vi "EMG_Contraction_Detection.vi"(4 "Triceps EMG signal (V)":dbl[](array[numeric]), 6 "Biceps EMG signal (V)":dbl[](array[numeric]), 7 "Biceps contraction threshold (V)":dbl, 9 "Biceps harder contraction threshold  (V)":dbl, 10 "Triceps harderd contraction threshold  (V)":dbl, 11 "Triceps contraction threshold  (V)":dbl) -> (0 "Triceps mean amplitude during contraction  (V)":dbl, 1 "Triceps hardly contracted?":bool, 2 "Triceps contracted?":bool, 3 "Biceps contracted?":bool, 5 "Biceps hardly contracted?":bool, 8 "Biceps mean amplitude during contraction  (V)":dbl)   [LabVIEW 2015]
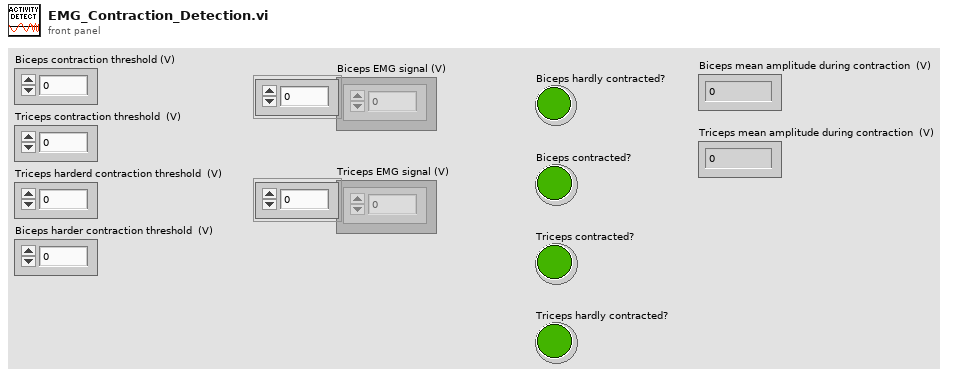
[diagram p1: front panel]
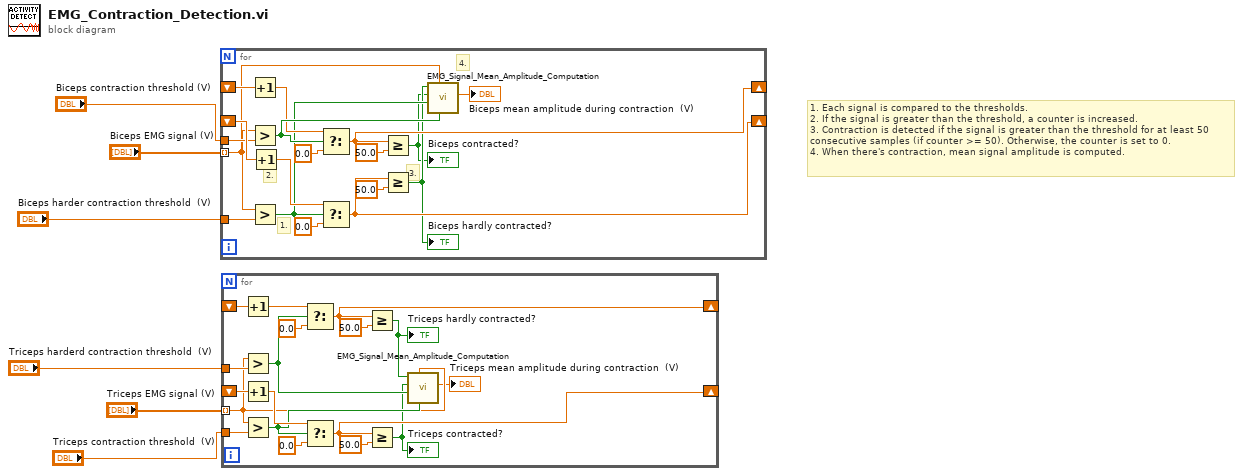
[diagram p0: block diagram]
diagram:
  # "1. Each signal is compared to the thresholds.\n2. If the signal is greater than the threshold, a counter is increased.\n3. Contraction is detected if the signal is greater than the threshold for at least 50\nconsecutive samples (if counter >= 50). Otherwise, the counter is set to 0.\n4. When there's contraction, mean signal amplitude is computed."
  n1 = for {
    tunnel: "Biceps EMG signal (V)" -> [w11] mode=indexing
    tunnel: "Biceps contraction threshold (V)" -> [w13]
    shift-right: [w15] -> _
    shift-left: _ -> [w24]
    shift-right: [w18] -> _
    shift-left: _ -> [w17]
    tunnel: "Biceps harder contraction threshold  (V)" -> [w16]
    # "4."
    # "3."
    # "2."
    # "1."
    n2 = Increment(x=w24) -> (x+1=w12:dbl)
    n3 = Greater?(x=w11, y=w13) -> (0:w14:bool)
    n4 = Greater?(x=w11, y=w16) -> (0:w10:bool)
    n5 = Increment(x=w17) -> (x+1=w21:dbl)
    n6 = Select(t=w12, s=w14, f=0.0) -> (s? t:f=w15:dbl)
    n7 = Select(t=w21, s=w10, f=0.0) -> (s? t:f=w18:dbl)
    n8 = Greater Or Equal?(x=w15, y=50.0) -> (x >= y?=w8:bool)
    "Biceps contracted?" <- w8
    n9 = Greater Or Equal?(x=w18, y=50.0) -> (x >= y?=w9:bool)
    "Biceps hardly contracted?" <- w9
    n10 = call "EMG_Signal_Mean_Amplitude_Computation.vi"("Greater than first threshold?"=w14, "EMG signal (V)"=w11, "Greater than second threshold?"=w10, "Contracted?"=w8, "Harder contracted?"=w9) -> ("Mean signal amplitude (V)"=→"Biceps mean amplitude during contraction  (V)":dbl)  [unwired: 6 in]
  }
  n11 = for {
    tunnel: "Triceps EMG signal (V)" -> [w26] mode=indexing
    tunnel: "Triceps contraction threshold  (V)" -> [w42]
    shift-right: [w38] -> _
    shift-left: _ -> [w40]
    shift-right: [w33] -> _
    shift-left: _ -> [w32]
    tunnel: "Triceps harderd contraction threshold  (V)" -> [w31]
    n12 = Increment(x=w32) -> (x+1=w36:dbl)
    n13 = Greater?(x=w26, y=w31) -> (0:w30:bool)
    n14 = Increment(x=w40) -> (x+1=w41:dbl)
    n15 = Greater?(x=w26, y=w42) -> (0:w29:bool)
    n16 = Select(t=w36, s=w30, f=0.0) -> (s? t:f=w33:dbl)
    n17 = Select(t=w41, s=w29, f=0.0) -> (s? t:f=w38:dbl)
    n18 = Greater Or Equal?(x=w33, y=50.0) -> (x >= y?=w27:bool)
    "Triceps hardly contracted?" <- w27
    n19 = Greater Or Equal?(x=w38, y=50.0) -> (x >= y?=w28:bool)
    "Triceps contracted?" <- w28
    n20 = call "EMG_Signal_Mean_Amplitude_Computation.vi"("Greater than first threshold?"=w29, "EMG signal (V)"=w26, "Greater than second threshold?"=w30, "Contracted?"=w28, "Harder contracted?"=w27) -> ("Mean signal amplitude (V)"=→"Triceps mean amplitude during contraction  (V)":dbl)  [unwired: 6 in]
  }
